vi "MAIN-DAQ-MK2.vi"() -> ()   [LabVIEW 2015]
uses:
  <vilib>/DAQmx/read.llb/DAQmx Read (Analog 1D DBL NChan 1Samp).vi
  <vilib>/Analysis/baseanly.llb/Mean (DBL).vi
  <vilib>/DAQmx/create/scale.llb/DAQmx Create Scale (Linear).vi
  <vilib>/DAQmx/create/channels.llb/DAQmx Create Channel (AI-Voltage-Basic).vi
  <vilib>/DAQmx/create/channels.llb/DAQmx Create Channel (AI-Temperature-Thermocouple).vi
  <vilib>/DAQmx/create/channels.llb/DAQmx Create Channel (AI-Pressure-Bridge-Two-Point-Linear).vi
  <vilib>/DAQmx/configure/timing.llb/DAQmx Timing (Sample Clock).vi
  <vilib>/DAQmx/configure/task.llb/DAQmx Configure Logging (TDMS).vi
  <vilib>/DAQmx/miscellaneous.llb/DAQmx Fill In Error Info.vi
  <resource>/objmgr/daqmx.rc
  <vilib>/Analysis/NI_AALBase.lvlib
panel:
  in  "Thrust Offset":dbl format="%0.2f"
  in  "Thrust Slope":dbl=1.0 format="%0.2f"
  in  "Pressure 2 Offset":dbl format="%0.2f"
  in  "Pressure 1 Offset":dbl format="%0.2f"
  in  "Pressure 2 Slope":dbl=1.0 format="%0.2f"
  in  "Pressure 1 Slope":dbl=1.0 format="%0.2f"
  in  "TC 4 Type":i32(ring)=10072 items=["J"=10072, "K"=10073, "N"=10077, "R"=10082, "S"=10085, "T"=10086, "B"=10047, "E"=10055]
  in  "TC 3 Type":i32(ring)=10072 items=["J"=10072, "K"=10073, "N"=10077, "R"=10082, "S"=10085, "T"=10086, "B"=10047, "E"=10055]
  in  "TC 2 Type":i32(ring)=10072 items=["J"=10072, "K"=10073, "N"=10077, "R"=10082, "S"=10085, "T"=10086, "B"=10047, "E"=10055]
  in  "TC 1 Type":i32(ring)=10072 items=["J"=10072, "K"=10073, "N"=10077, "R"=10082, "S"=10085, "T"=10086, "B"=10047, "E"=10055]
  out "?":dbl
  out "?":dbl
  out "?":dbl
  out "?":dbl
  out "?":dbl
  out "Thrust":dbl(slide) scale=0.0..500.0
  out "TC 4":dbl(slide) scale=0.0..1200.0
  out "TC 3":dbl(slide) max=20.0 scale=0.0..1200.0
  out "TC 2":dbl(slide) scale=0.0..1200.0
  out "TC 1":dbl(slide) scale=0.0..1200.0
  out "?":dbl
  out "?":dbl
  out "Pressure 2":dbl(knob) scale=0.0..800.0
  out "Pressure 1":dbl(knob) scale=0.0..2000.0
  in  "Pressure 2":tag
  in  "Pressure 1":tag
  in  "TC 4":tag
  in  "TC 3":tag
  in  "TC 2":tag
  in  "TC 1":tag
  in  "Load Cell":tag
  in  "?":bool
  in  "?":string="Job 1 - Day 1"
  in  "?":bool
  out "Number of Sensors":sgl
  in  "?":bool
  in  "Samples Per Update":dbl=100.0
  out "Current Group":string="Group 0"
  in  "Sampling Rate [Hz]":i32=10000
  in  "Logging Mode":i32(ring)=15842 items=["Off"=10231, "Log"=15844, "Log and Read"=15842]
  in  "File Path":path=path "test1.tdms"
  # "Data Logging Settings"
  # "Sensor Settings"
  # "Sampling Settings"
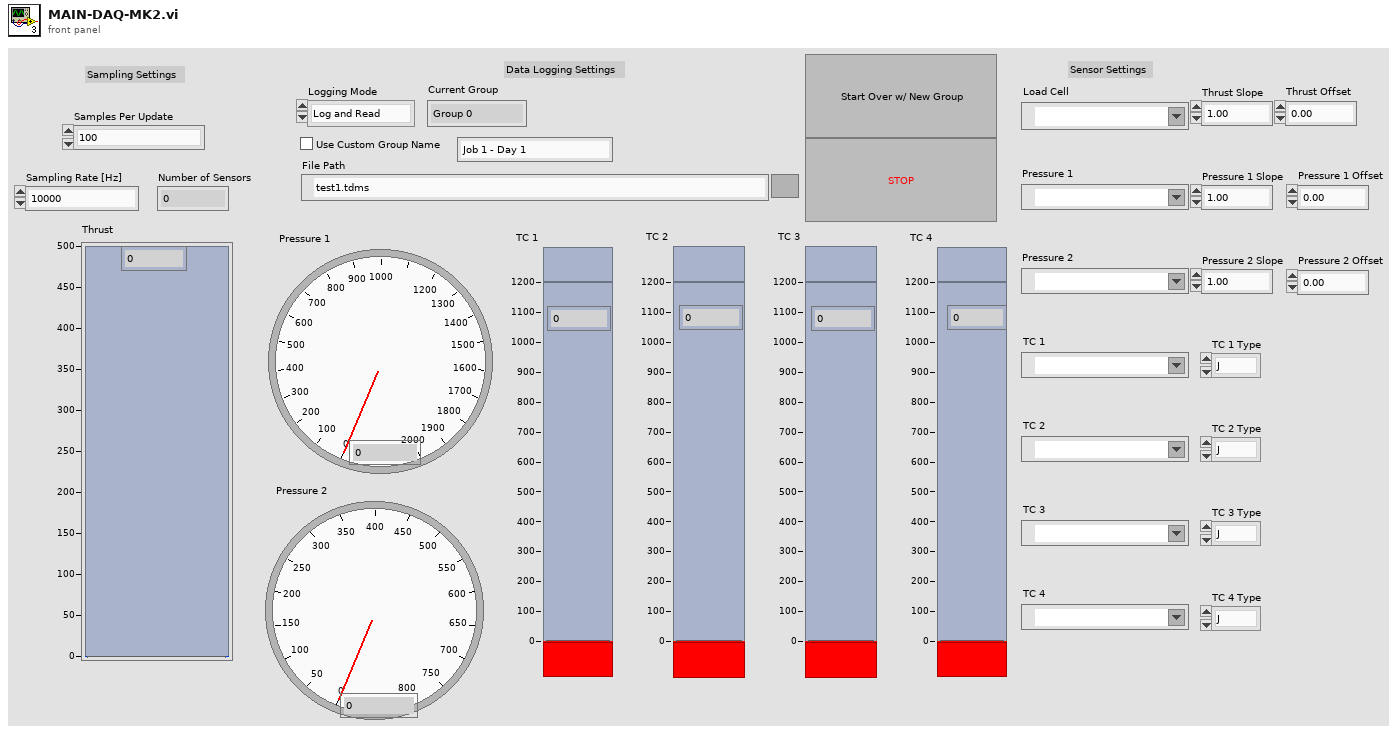
[diagram p1: front panel]
types:
  T1 = enum16{"open", "open or create", "create or replace", "create", "open (read-only)"}
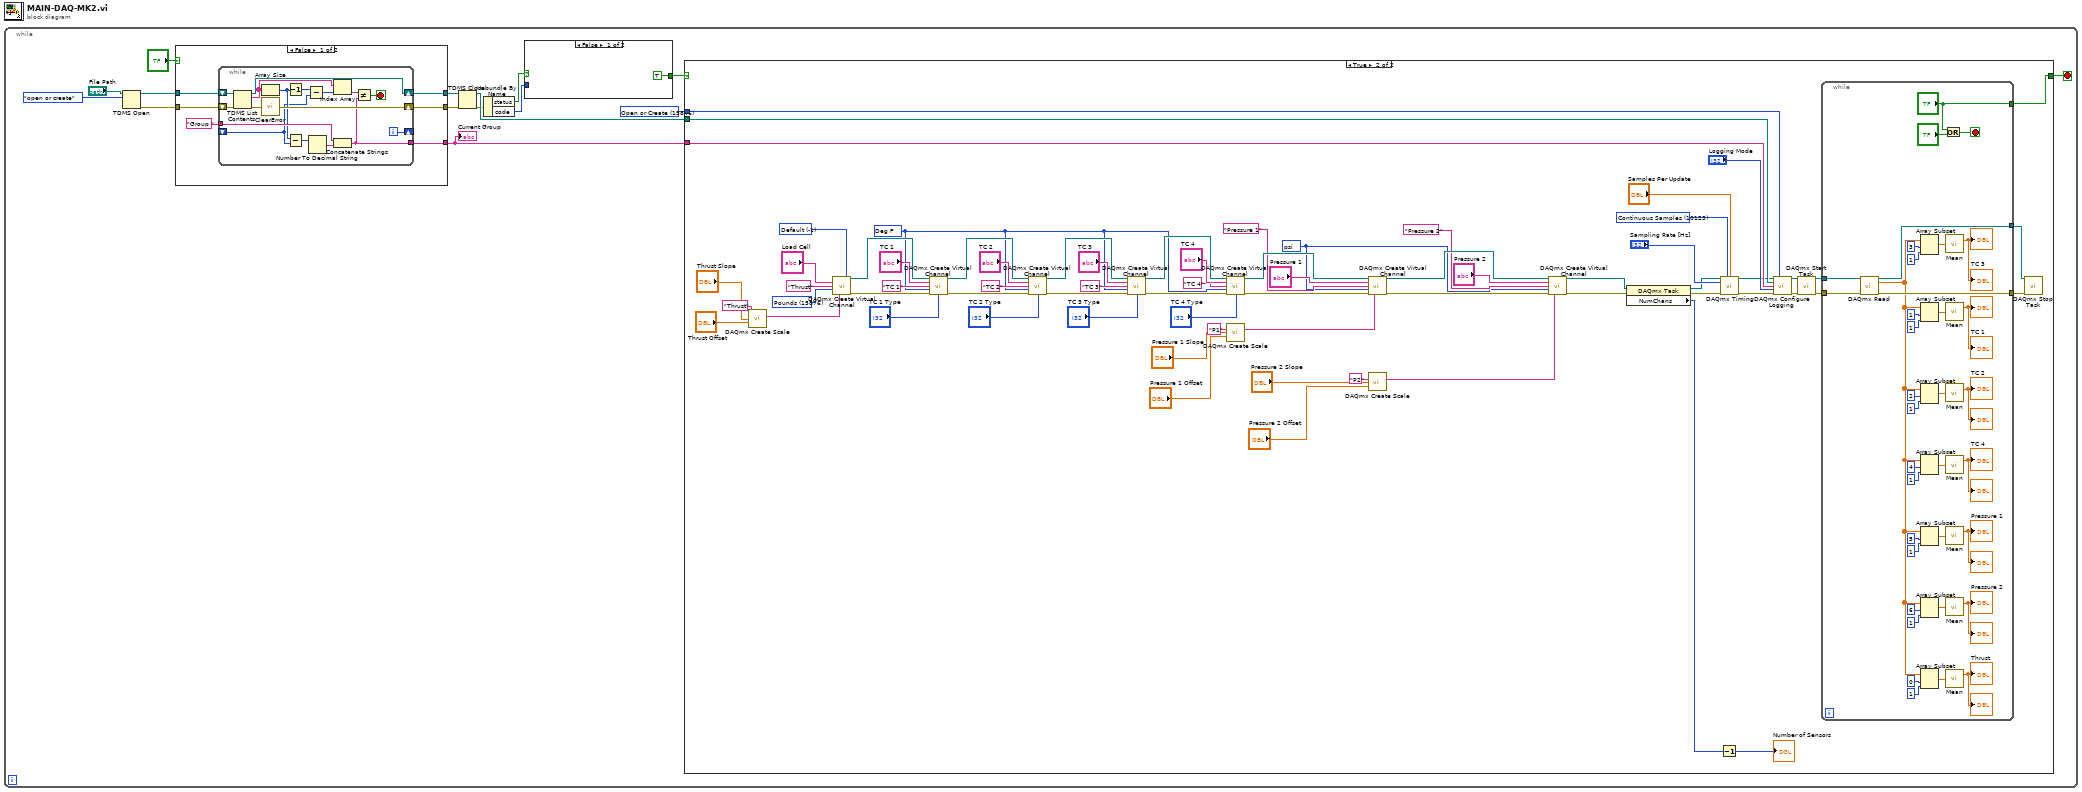
[diagram p0: block diagram]
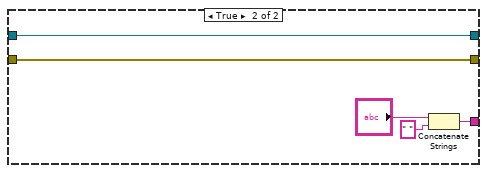
[diagram p2: hidden frame]
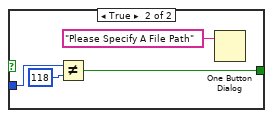
[diagram p3: hidden frame]
diagram:
  n1 = while {
    stop <- w6 stop-if-true
    w15 = 15846 items=["Open"=10437, "Open or Create"=15846, "Create or Replace"=15847, "Create"=15848] ("operation")
    n2 = TDMS Open(10:T1."open or create" ("operation (0:open)"), 11:"File Path") -> (0:w4:errorcluster, 3:w5:refnum<k34>)  [unwired: 5 in]
    n3 = case shown="False" "?" {
      tunnel: [w18 w41] -> w1
      tunnel: w5 -> [w21 w40]
      tunnel: w4 -> [w20 w39]
      tunnel: [w17 w40] -> w3
      tunnel: [w16 w39] -> w2
      frame False {
        n4 = while {
          shift-right: [w37] -> w17
          shift-left: w21 -> [w38]
          shift-right: [w35] -> w16
          shift-left: w20 -> [w36]
          tunnel: "Group " -> [w33]
          tunnel: [w30] -> w18
          shift-right: [w26] -> _
          shift-left: _ -> [w24]
          i -> [w26]
          stop <- w31 stop-if-true
          n5 = TDMS List Contents(4:w36, 7:w38) -> (0:w22:errorcluster, 2:w29:string[], 3:w37:refnum<k34>)  [unwired: 1 in, 1 out]
          n6 = Array Size(array=w29) -> (size(s)=w25:i32)
          n7 = call <vilib>:"ClearError.vi"("error in (no error)"=w22) -> ("error out"=w35:errorcluster)
          n8 = Decrement(x=w25) -> (x-1=w27:i32)
          n9 = Subtract(x=w25, y=w24) -> (x-y=w23:i32)
          n10 = Subtract(x=w27, y=w24) -> (x-y=w28:i32)
          n11 = Number To Decimal String(number=w23) -> (decimal integer string=w34:string)  [unwired: 1 in]
          n12 = Index Array(array=w29, index=w28) -> (element=w32:string)
          n13 = Concatenate Strings(w33, w34) -> (w30:string)
          n14 = Not Equal?(x=w32, y=w30) -> (x != y?=w31:bool)
        }
      }
      frame True {
        n15 = Concatenate Strings("?", " ") -> (w41:string)
      }
    }
    "Current Group" <- w1
    n16 = TDMS Close(8:w2, 11:w3) -> (0:w11:errorcluster, 3:w13:path)
    n17 = Unbundle By Name(w11) -> ("status"=w10:bool, "code"=w9:i32)
    n18 = case shown="False" w10 {
      tunnel: w9 -> [_ w47]
      tunnel: [TRUE w46] -> w8
      frame False {
      }
      frame True {
        n19 = Not Equal?(x=w47, y=118) -> (x != y?=w46:bool)
        n20 = One Button Dialog(message="Please Specify A File Path") -> ()  [unwired: 1 in, 1 out]
      }
    }
    n21 = case shown="True" w8 {
      selector: w8 -> [w49 _]
      tunnel: w15 -> [_ w112]
      tunnel: w13 -> [_ w111]
      tunnel: w1 -> [_ w110]
      tunnel: [w49 w100] -> w6
      frame False {
      }
      frame True {
        w61 = -1 items=["Default"=-1, "RSE"=10083, "NRSE"=10078, "Differential"=10106, "Pseudodifferential"=12529] ("input terminal configuration")
        w67 = 15879 items=["Pascals"=10081, "psi"=15879, "bar"=15880, "From Custom Scale"=10065] ("units")
        w68 = 10144 items=["Deg C"=10143, "Deg F"=10144, "Kelvins"=10325, "Deg R"=10145, "From Custom Scale"=10065] ("units")
        w98 = 15876 items=["Newtons"=15875, "Pounds"=15876, "From Custom Scale"=10065] ("units")
        w109 = 10123 items=["Finite Samples"=10178, "Continuous Samples"=10123, "Hardware Timed Single Point"=12522] ("sample mode")
        n22 = call-poly <vilib>:"DAQmx Create Scale.vi"("name"="Thrust", "slope"="Thrust Slope", "y-intercept"="Thrust Offset") -> ("scale out"=w62:tag)  [unwired: 11 in, 1 out]
        n23 = call-poly <vilib>:"DAQmx Create Virtual Channel.vi"("input terminal configuration"=w61, "physical channels"="Load Cell", "name to assign"="Thrust", "units"=w98, "custom scale name"=w62) -> ("task out"=w95:refnum<k21>, "error out"=w88:errorcluster)  [unwired: 9 in]
        n24 = call-poly <vilib>:"DAQmx Create Virtual Channel.vi"("task in"=w95, "physical channels"="TC 1", "name to assign"="TC 1", "units"=w68, "error in"=w88, "thermocouple type"="TC 1 Type") -> ("task out"=w94:refnum<k21>, "error out"=w87:errorcluster)  [unwired: 8 in]
        n25 = call-poly <vilib>:"DAQmx Create Virtual Channel.vi"("task in"=w94, "physical channels"="TC 2", "name to assign"="TC 2", "units"=w68, "error in"=w87, "thermocouple type"="TC 2 Type") -> ("task out"=w93:refnum<k21>, "error out"=w86:errorcluster)  [unwired: 8 in]
        n26 = call-poly <vilib>:"DAQmx Create Virtual Channel.vi"("task in"=w93, "physical channels"="TC 3", "name to assign"="TC 3", "units"=w68, "error in"=w86, "thermocouple type"="TC 3 Type") -> ("task out"=w92:refnum<k21>, "error out"=w85:errorcluster)  [unwired: 8 in]
        n27 = call-poly <vilib>:"DAQmx Create Virtual Channel.vi"("task in"=w92, "physical channels"="TC 4", "name to assign"="TC 4", "units"=w68, "error in"=w85, "thermocouple type"="TC 4 Type") -> ("task out"=w91:refnum<k21>, "error out"=w84:errorcluster)  [unwired: 8 in]
        n28 = call-poly <vilib>:"DAQmx Create Scale.vi"("name"="P1", "slope"="Pressure 1 Slope", "y-intercept"="Pressure 1 Offset") -> ("scale out"=w60:tag)  [unwired: 11 in, 1 out]
        n29 = call-poly <vilib>:"DAQmx Create Virtual Channel.vi"("task in"=w91, "physical channels"="Pressure 1", "name to assign"="Pressure 1", "units"=w67, "error in"=w84, "custom scale name"=w60) -> ("task out"=w90:refnum<k21>, "error out"=w83:errorcluster)  [unwired: 8 in]
        n30 = call-poly <vilib>:"DAQmx Create Scale.vi"("name"="P2", "slope"="Pressure 2 Slope", "y-intercept"="Pressure 2 Offset") -> ("scale out"=w59:tag)  [unwired: 11 in, 1 out]
        n31 = call-poly <vilib>:"DAQmx Create Virtual Channel.vi"("task in"=w90, "physical channels"="Pressure 2", "name to assign"="Pressure 2", "units"=w67, "error in"=w83, "custom scale name"=w59) -> ("task out"=w89:refnum<k21>, "error out"=w75:errorcluster)  [unwired: 8 in]
        n32 = property class="DAQmx Task"(reference=w89, error in=w75) -> (reference out=w103:refnum<k21>, error out=w102:errorcluster, "NumChans"=w101:u32)
        n33 = Decrement(x=w101) -> (x-1=→"Number of Sensors":u32)
        n34 = call-poly <vilib>:"DAQmx Timing.vi"("task/channels in"=w103, "sample mode"=w109, "samples per channel"="Samples Per Update", "rate"="Sampling Rate [Hz]", "error in"=w102) -> ("task out"=w104:refnum<k21>, "error out"=w113:errorcluster)  [unwired: 9 in]
        n35 = call-poly <vilib>:"DAQmx Configure Logging.vi"("task/channels in"=w104, "operation"=w112, "file path"=w111, "group name"=w110, "logging mode"="Logging Mode", "error in"=w113) -> ("task out"=w117:refnum<k21>, "error out"=w116:errorcluster)  [unwired: 8 in]
        n36 = call <vilib>:"DAQmx Start Task.vi"("task/channels in"=w117, "error in"=w116) -> ("task out"=w108:refnum<k21>, "error out"=w107:errorcluster)  [unwired: 12 in]
        n37 = while {
          tunnel: w108 -> [w153]
          tunnel: w107 -> [w152]
          tunnel: [w151] -> w106
          tunnel: [w150] -> w105
          tunnel: ["?"] -> w100
          stop <- w118 stop-if-true
          n38 = call-poly <vilib>:"DAQmx Read.vi"("task/channels in"=w153, "error in"=w152) -> ("task out"=w151:refnum<k21>, "data"=w140:dbl[], "error out"=w150:errorcluster)  [unwired: 11 in]
          n39 = Array Subset(array=w140, index=3, length=1) -> (w130:dbl[])
          n40 = Array Subset(array=w140, index=1, length=1) -> (w132:dbl[])
          n41 = Array Subset(array=w140, index=2, length=1) -> (w131:dbl[])
          n42 = Array Subset(array=w140, index=4, length=1) -> (w129:dbl[])
          n43 = Array Subset(array=w140, index=5, length=1) -> (w128:dbl[])
          n44 = Array Subset(array=w140, index=6, length=1) -> (w127:dbl[])
          n45 = Array Subset(array=w140, index=0, length=1) -> (w126:dbl[])
          n46 = Or(x="?", y="?") -> (x .or. y?=w118:bool)
          n47 = call-poly <vilib>:"Mean.vi"("X"=w130) -> ("mean"=→"TC 3" →"?":dbl)  [unwired: 1 out]
          n48 = call-poly <vilib>:"Mean.vi"("X"=w132) -> ("mean"=→"TC 1" →"?":dbl)  [unwired: 1 out]
          n49 = call-poly <vilib>:"Mean.vi"("X"=w131) -> ("mean"=→"TC 2" →"?":dbl)  [unwired: 1 out]
          n50 = call-poly <vilib>:"Mean.vi"("X"=w129) -> ("mean"=→"TC 4" →"?":dbl)  [unwired: 1 out]
          n51 = call-poly <vilib>:"Mean.vi"("X"=w128) -> ("mean"=→"Pressure 1" →"?":dbl)  [unwired: 1 out]
          n52 = call-poly <vilib>:"Mean.vi"("X"=w127) -> ("mean"=→"Pressure 2" →"?":dbl)  [unwired: 1 out]
          n53 = call-poly <vilib>:"Mean.vi"("X"=w126) -> ("mean"=→"Thrust" →"?":dbl)  [unwired: 1 out]
        }
        n54 = call <vilib>:"DAQmx Stop Task.vi"("task/channels in"=w106, "error in"=w105) -> ()  [unwired: 12 in, 2 out]
      }
    }
  }
